vi "FpgaLink_Close.vi"(8 "error in (no error)":errorcluster, 11 "handle":i64) -> (0 "error out":errorcluster)   [LabVIEW 2011]
doc: "Close the connection to the FPGALink device."
uses:
  libfpgalink.dll
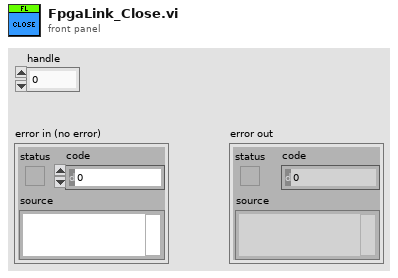
[diagram p1: front panel]
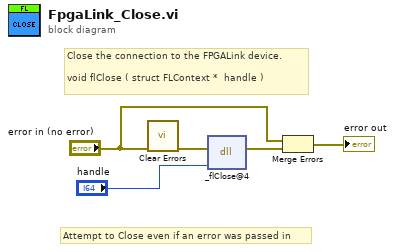
[diagram p0: block diagram]
diagram:
  # "Attempt to Close even if an error was passed in"
  # "Close the connection to the FPGALink device.\n\nvoid flClose\t(\tstruct FLContext * \thandle\t)"
  n1 = call <vilib>:"Clear Errors.vi"("error in (no error)"="error in (no error)") -> ("error out"=w4:errorcluster)  [unwired: 6 in]
  n2 = dll-call lib="libfpgalink.dll" fn="_flClose@4"(error in=w4, "handle"="handle") -> (error out=w3:errorcluster)  [unwired: 4 in, 1 out]
  n3 = Merge Errors("error in (no error)", w3) -> (→"error out":errorcluster)
